vi "AAroute.vi"() -> ()   [LabVIEW 2014]
uses:
  <vilib>/Utility/sysdir.llb/System Directory Type.ctl
  <vilib>/httpClient/LabVIEWHTTPClient.lvlib
panel:
  out "time":string
  in  "저장 경로":path
  out "Distance":string="0"
  in  "?":bool
  in  "정규식 5":string
  in  "정규식 4":string
  in  "정규식 3":string
  in  "?":bool
  in  "?":bool
  out "x fmc 플랜":string
  out "FMS 플랜":string
  in  "Destination":string
  in  "departure":string
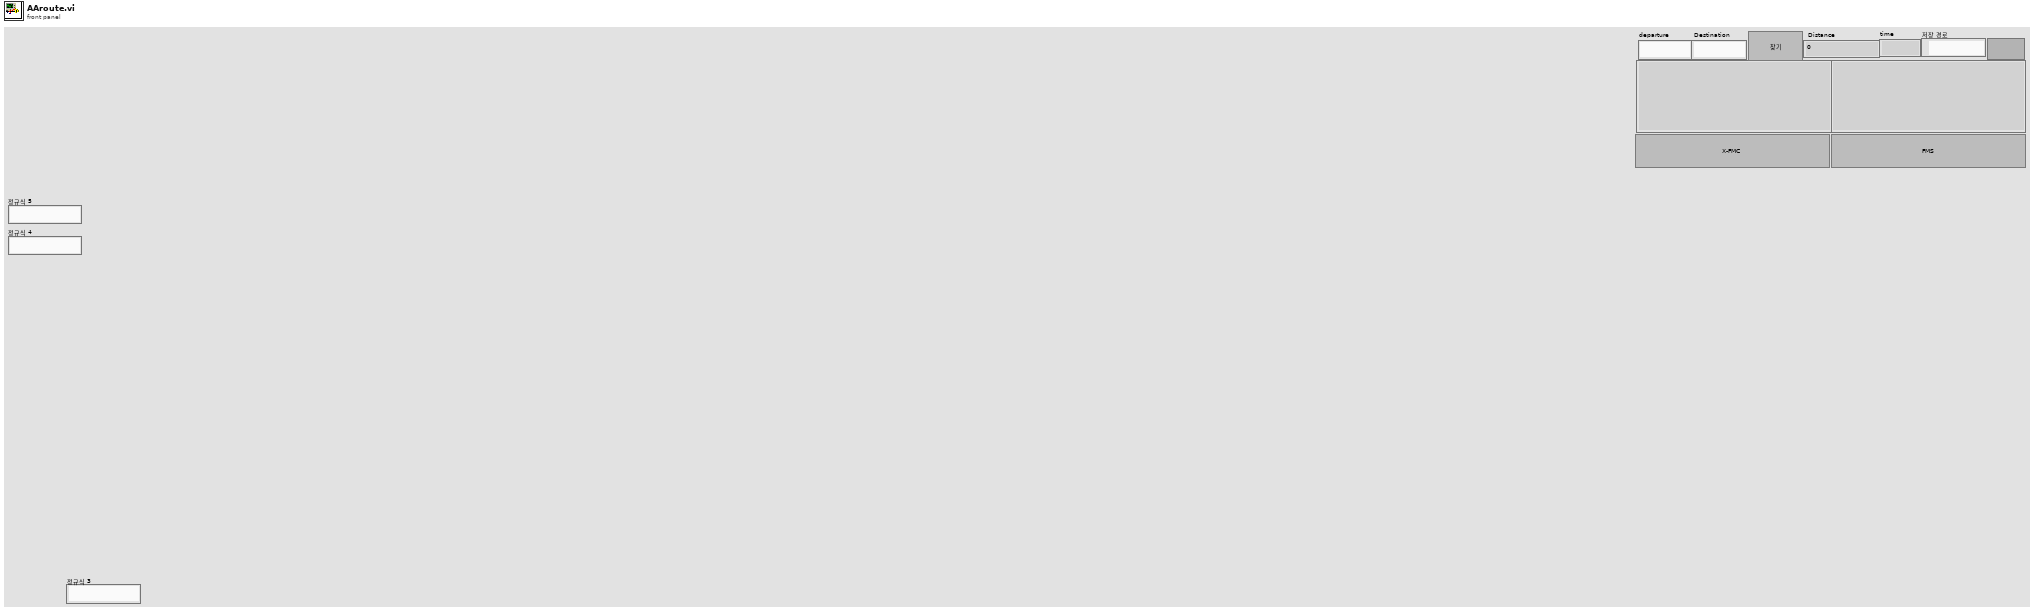
[diagram p1: front panel]
types:
  T1 = enum16{"open", "replace", "create", "open or create", "replace or create", "replace or create with confirmation"}
  T2 = typedef "System Directory Type.ctl" = i32
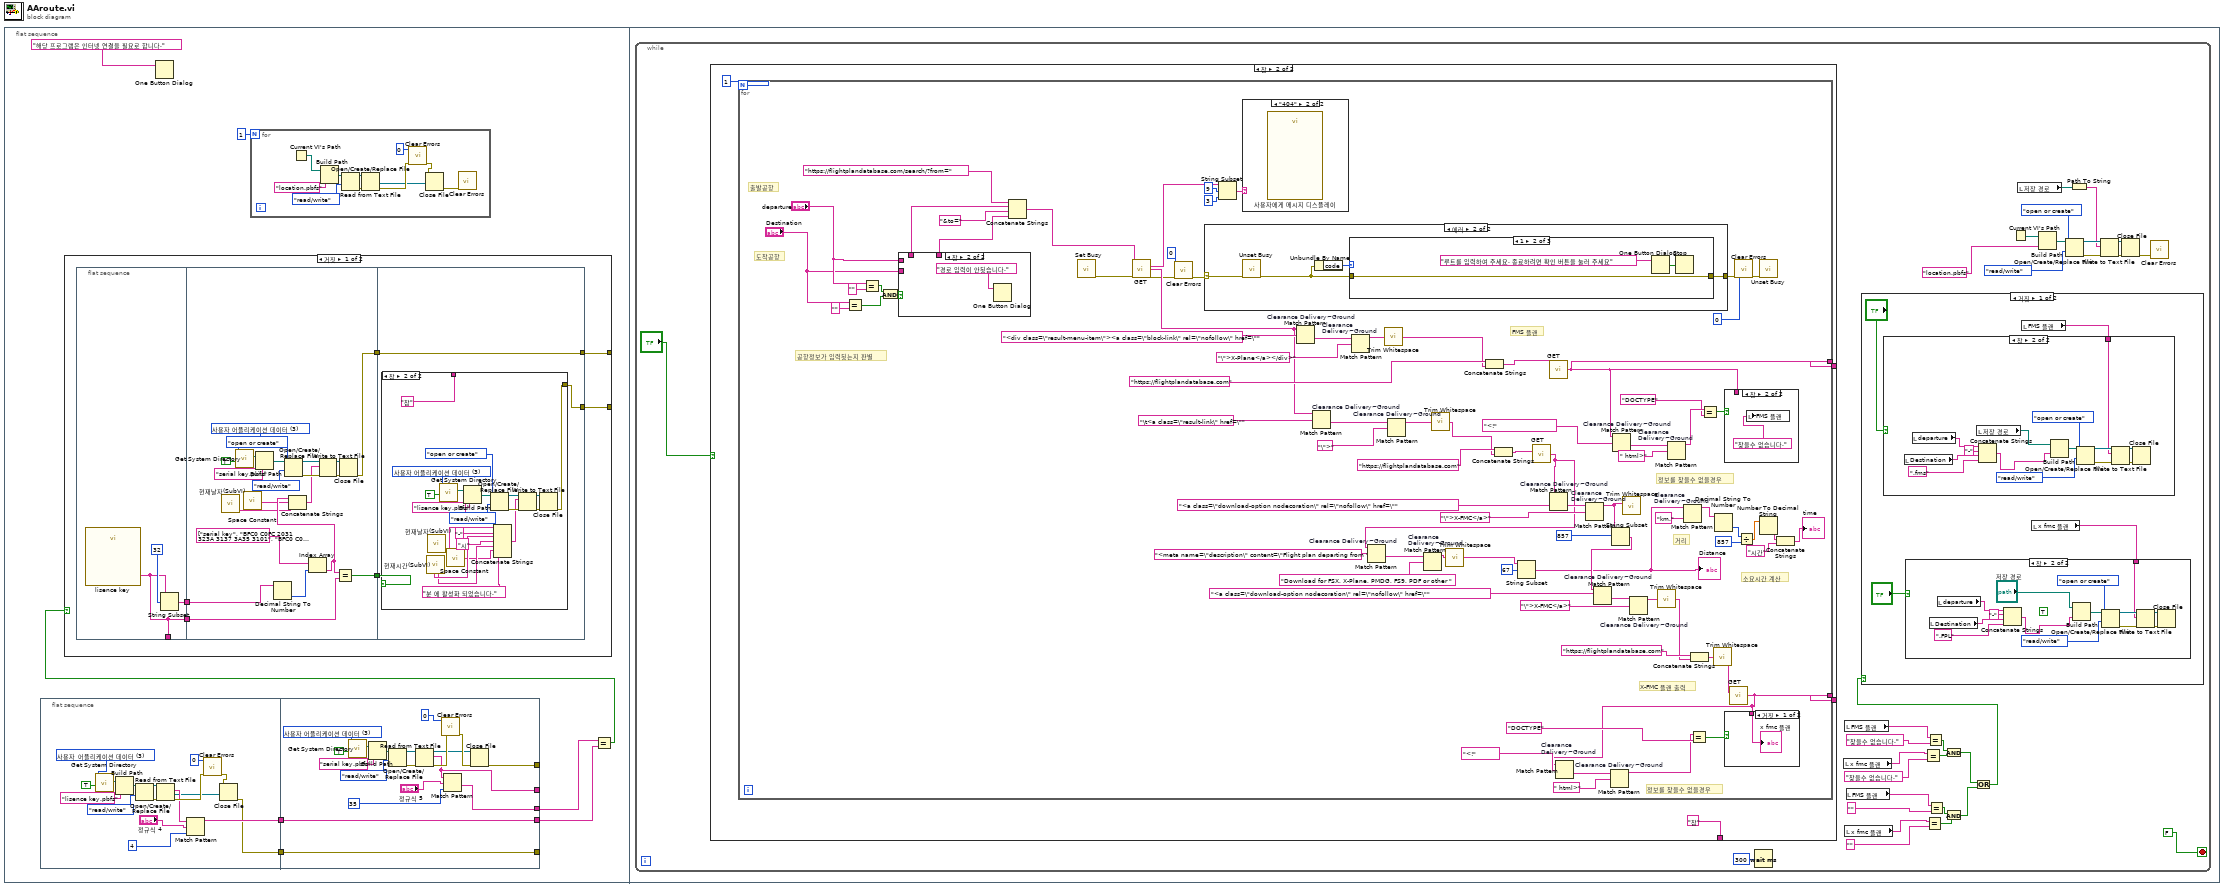
[diagram p0: block diagram]
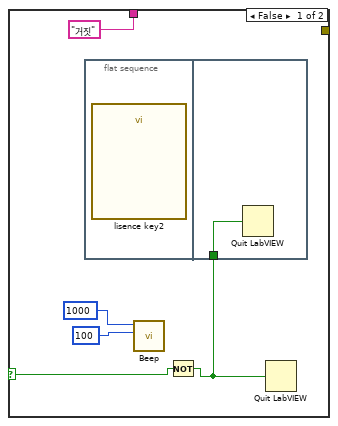
[diagram p2: hidden frame]
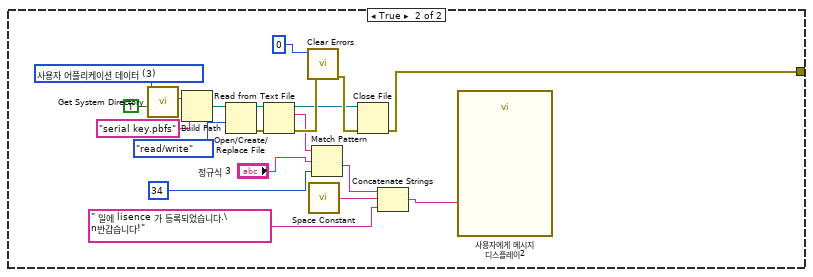
[diagram p3: hidden frame]
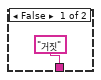
[diagram p7: hidden frame]
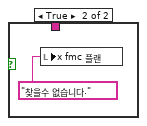
[diagram p9: hidden frame]
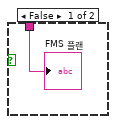
[diagram p10: hidden frame]
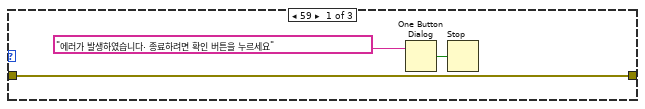
[diagram p13: hidden frame]
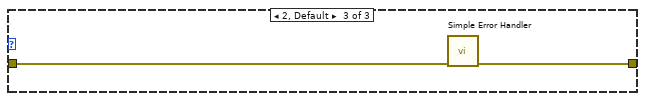
[diagram p14: hidden frame]
diagram:
  n1 = flat-sequence {
    frame #0 {
      n2 = flat-sequence {
        tunnel: [w20] -> w7
        tunnel: [w19] -> w6
        tunnel: [w42] -> w4
        tunnel: w7 -> [w42]
        tunnel: [w40] -> w5
        tunnel: [w36] -> _
        tunnel: [w38] -> _
        tunnel: w6 -> [w38]
        tunnel: [w37] -> _
        frame #0 {
          w25 = T2 3 items=["사용자 홈"=0, "사용자 데스크탑"=1, "사용자 문서"=2, "사용자 어플리케이션 데이터"=3, "사용자 환경"=4, "사용자 임시"=5, "퍼블릭 문서"=6, "퍼블릭 어플리케이션 데이터"=7, "퍼블릭 환경"=8, "퍼블릭 캐시"=13, "시스템 코어 라이브러리"=9, "시스템 설치된 라이브러리"=10, "어플리케이션 파일"=11, "부팅 볼륨 루트"=12] ("system directory type")
          n3 = call <vilib>:"Get System Directory.vi"("create directory if not found? (F)"=TRUE, "system directory type"=w25) -> ("system directory"=w24:path)  [unwired: 9 in]
          n4 = Build Path(base path=w24, name or relative path="lisence key.pbfs" ("이름 또는 상대 경로")) -> (appended path=w23:path)
          n5 = Open/Create/Replace File(file path (use dialog)=w23, access (0:read/write)=enum16{"read/write", "read-only", "write-only"}."read/write" ("접근(0:읽기/쓰기)")) -> (refnum out=w29:refnum<file>, error out=w28:errorcluster)  [unwired: 4 in, 1 out]
          n6 = Read from Text File(file (use dialog)=w29, error in=w28) -> (refnum out=w30:refnum<file>, text=w31:string, error out=w33:errorcluster)  [unwired: 2 in, 1 out]
          n7 = Match Pattern(string=w31, regular expression="정규식 4", offset (0)=4 ("오프셋(0) 2")) -> (before substring=w20:string)  [unwired: 3 out]
          n8 = call <vilib>:"Clear Errors.vi"("error in (no error)"=w33, "specific error code to clear (0: all)"=0) -> ("error out"=w34:errorcluster)  [unwired: 4 in, 1 out]
          n9 = Close File(refnum=w30, error in=w34) -> (error out=w19:errorcluster)  [unwired: 1 out]
        }
        frame #1 {
          w48 = T2 3 items=["사용자 홈"=0, "사용자 데스크탑"=1, "사용자 문서"=2, "사용자 어플리케이션 데이터"=3, "사용자 환경"=4, "사용자 임시"=5, "퍼블릭 문서"=6, "퍼블릭 어플리케이션 데이터"=7, "퍼블릭 환경"=8, "퍼블릭 캐시"=13, "시스템 코어 라이브러리"=9, "시스템 설치된 라이브러리"=10, "어플리케이션 파일"=11, "부팅 볼륨 루트"=12] ("system directory type")
          n10 = call <vilib>:"Get System Directory.vi"("create directory if not found? (F)"=TRUE, "system directory type"=w48) -> ("system directory"=w49:path)  [unwired: 9 in]
          n11 = Build Path(base path=w49, name or relative path="serial key.pbfs" ("이름 또는 상대 경로")) -> (appended path=w50:path)
          n12 = Open/Create/Replace File(file path (use dialog)=w50, access (0:read/write)=enum16{"read/write", "read-only", "write-only"}."read/write" ("접근(0:읽기/쓰기)")) -> (refnum out=w44:refnum<file>, error out=w45:errorcluster)  [unwired: 4 in, 1 out]
          n13 = Read from Text File(file (use dialog)=w44, error in=w45) -> (refnum out=w43:refnum<file>, text=w36:string, error out=w52:errorcluster)  [unwired: 2 in, 1 out]
          n14 = call <vilib>:"Clear Errors.vi"("error in (no error)"=w52, "specific error code to clear (0: all)"=0) -> ("error out"=w53:errorcluster)  [unwired: 4 in, 1 out]
          n15 = Match Pattern(string=w36, regular expression="정규식 5", offset (0)=35 ("오프셋(0)")) -> (after substring=w40:string)  [unwired: 3 out]
          n16 = Close File(refnum=w43, error in=w53) -> (error out=w37:errorcluster)  [unwired: 1 out]
        }
      }
      n17 = One Button Dialog(message="해당 프로그램은 인터넷 연결을 필요로 합니다." ("메시지")) -> ()  [unwired: 1 in, 1 out]
      n18 = for {
        N: 1 -> [_]
        n19 = Current VI's Path() -> (path=w9:path)
        n20 = Build Path(base path=w9, name or relative path="location.pbfs" ("이름 또는 상대 경로")) -> (appended path=w10:path)
        n21 = Open/Create/Replace File(file path (use dialog)=w10, access (0:read/write)=enum16{"read/write", "read-only", "write-only"}."read/write" ("접근(0:읽기/쓰기)")) -> (refnum out=w14:refnum<file>, error out=w13:errorcluster)  [unwired: 4 in, 1 out]
        n22 = Read from Text File(file (use dialog)=w14, error in=w13) -> (refnum out=w15:refnum<file>, error out=w16:errorcluster)  [unwired: 2 in, 2 out]
        n23 = call <vilib>:"Clear Errors.vi"("error in (no error)"=w16, "specific error code to clear (0: all)"=0) -> ("error out"=w17:errorcluster)  [unwired: 4 in, 1 out]
        n24 = Close File(refnum=w15, error in=w17) -> (error out=w8:errorcluster)  [unwired: 1 out]
        n25 = call <vilib>:"Clear Errors.vi"("error in (no error)"=w8) -> ()  [unwired: 5 in, 2 out]
      }
      n26 = Equal?(x=w5, y=w4) -> (x = y?=w3:bool)
      n27 = case shown="거짓" w3 {
        tunnel: [w56 w115] -> _
        tunnel: [w55 _] -> _
        frame False {
          n28 = flat-sequence {
            tunnel: [w62] -> w60
            tunnel: [w61] -> w59
            tunnel: [w61] -> _
            tunnel: w60 -> [w84]
            tunnel: [w81] -> w58
            tunnel: w59 -> [w82]
            tunnel: [w65] -> w57
            tunnel: w58 -> [w87]
            tunnel: [w86] -> w56
            tunnel: w57 -> [w85]
            tunnel: [w85] -> w55
            frame #0 {
              n29 = call "lisence key"() -> ("lisence key"=w61:string)  [unwired: 17 in, 2 out]
              n30 = String Subset(string=w61, offset (0)=32 ("오프셋(0)")) -> (substring=w62:string)  [unwired: 1 in]
            }
            frame #1 {
              w74 = T2 3 items=["사용자 홈"=0, "사용자 데스크탑"=1, "사용자 문서"=2, "사용자 어플리케이션 데이터"=3, "사용자 환경"=4, "사용자 임시"=5, "퍼블릭 문서"=6, "퍼블릭 어플리케이션 데이터"=7, "퍼블릭 환경"=8, "퍼블릭 캐시"=13, "시스템 코어 라이브러리"=9, "시스템 설치된 라이브러리"=10, "어플리케이션 파일"=11, "부팅 볼륨 루트"=12] ("system directory type")
              n31 = call "현재날자(SubVI).vi"() -> ("월,일 을 문자열로"=w69:string)  [unwired: 5 in, 6 out]
              n32 = call <vilib>:"Get System Directory.vi"("create directory if not found? (F)"=TRUE, "system directory type"=w74) -> ("system directory"=w73:path)  [unwired: 9 in]
              n33 = call <vilib>:"Space Constant.vi"() -> ("String"=w68:string)
              n34 = Build Path(base path=w73, name or relative path="serial key.pbfs" ("이름 또는 상대 경로")) -> (appended path=w72:path)
              n35 = Decimal String To Number(string=w84) -> (number=w83:i32)  [unwired: 2 in, 1 out]
              n36 = Open/Create/Replace File(file path (use dialog)=w72, operation (0:open)=T1."open or create" ("동작(0:open)"), access (0:read/write)=enum16{"read/write", "read-only", "write-only"}."read/write" ("접근(0:읽기/쓰기)")) -> (refnum out=w80:refnum<file>, error out=w79:errorcluster)  [unwired: 3 in, 1 out]
              n37 = Index Array(array=string[] ["serial key", "BFC0 C0FC 2031 323A 3137 3A35 3101", "BFC0 C0FC 2031 323A 3138 3A30 3902", "BFC0 C0FC 2031 323A 3139 3A30 3903", "BFC0 C0FC 2031 323A 3230 3A30 3904", "BFC0 C0FC 2031 323A 3231 3A30 3905", "BFC0 C0FC 2031 323A 3232 3A30 3906", "BFC0 C0FC 2031 323A 3233 3A30 3907", "BFC0 C0FC 2031 323A 3234 3A30 3908", "BFC0 C0FC 2031 323A 3235 3A30 3909", "BFC0 C0FC 2031 323A 3236 3A30 3910", "BFC0 C0FC 2031 323A 3237 3A30 3911", "BFC0 C0FC 2031 323A 3238 3A30 3912", "BFC0 C0FC 2031 323A 3239 3A30 3913", "BFC0 C0FC 2031 323A 3036 3A33 3214", "BFC0 C0FC 2031 323A 3037 3A33 3215", "BFC0 C0FC 2031 323A 3038 3A33 3216", "BFC0 C0FC 2031 323A 3038 3A33 3217", "BFC0 C0FC 2031 323A 3039 3A33 3218", "BFC0 C0FC 2031 323A 3039 3A35 3019", "BFC0 C0FC 2031 323A 3130 3A35 3020", "BFC0 C0FC 2031 323A 3131 3A35 3121", "BFC0 C8C4 2031 313A 3536 3A33 3222", "BFC0 C8C4 2031 313A 3537 3A33 3223", "BFC0 C8C4 2031 313A 3538 3A33 3224", "BFC0 C8C4 2031 313A 3539 3A33 3225", "BFC0 C0FC 2031 323A 3030 3A33 3226", "BFC0 C0FC 2031 323A 3031 3A33 3227", "BFC0 C0FC 2031 323A 3032 3A33 3228", "BFC0 C0FC 2031 323A 3033 3A33 3229", "BFC0 C0FC 2031 323A 3034 3A33 3230", "BFC0 C0FC 2031 323A 3035 3A33 3231", "BFC0 C0FC 2031 323A 3036 3A33 3232", "BFC0 C0FC 2031 323A 3037 3A33 3233", "BFC0 C0FC 2031 323A 3038 3A33 3234", "BFC0 C0FC 2033 3A34 373A 3031 0035 ", "BFC0 C0FC 2033 3A34 383A 3234 0036", "BFC0 C0FC 2033 3A34 393A 3132 0037", "BFC0 C0FC 2033 3A35 303A 3534 0038", "BFC0 C0FC 2033 3A35 313A 3231 0039 ", "BFC0 C0FC 2033 3A35 323A 3333 0040 ", "BFC0 C0FC 2033 3A35 333A 3030 0041", "BFC0 C0FC 2033 3A35 343A 3432 0042", "BFC0 C0FC 2033 3A35 353A 3431 0043", "BFC0 C0FC 2033 3A35 363A 3131 0044", "BFC0 C0FC 2033 3A35 373A 3239 0045", "BFC0 C0FC 2033 3A35 383A 3539 0046", "BFC0 C0FC 2033 3A35 393A 3533 0047", "BFC0 C0FC 2034 3A30 303A 3430 0048 "] ("출력 배열"), index=w83) -> (element=w70:string)
              n38 = Concatenate Strings(w70, w68, w69) -> (w71:string)
              n39 = Write to Text File(file (use dialog)=w80, text=w71, error in=w79) -> (refnum out=w77:refnum<file>, error out=w78:errorcluster)  [unwired: 1 in, 1 out]
              n40 = Equal?(x=w70, y=w82) -> (x = y?=w81:bool)
              n41 = Close File(refnum=w77, error in=w78) -> (error out=w65:errorcluster)  [unwired: 1 out]
            }
            frame #2 {
              n42 = case shown="참" w87 {
                selector: w87 -> [w90 _]
                tunnel: ["거짓" "참"] -> _
                tunnel: [_ w94] -> w86
                frame False {
                  n43 = flat-sequence {
                    tunnel: w91 -> [w93]
                    frame #0 {
                      n44 = call "lisence key2"() -> ()  [unwired: 10 in, 2 out]
                    }
                    frame #1 {
                      n45 = Quit LabVIEW(quit? (T)=w93) -> ()
                    }
                  }
                  n46 = call <vilib>:"Beep.vi"("duration (msec)"=u32 100, "frequency (Hz)"=u32 1000) -> ()  [unwired: 10 in]
                  n47 = Not(x=w90) -> (.not. x?=w91:bool)
                  n48 = Quit LabVIEW(quit? (T)=w91) -> ()
                }
                frame True {
                  w110 = T2 3 items=["사용자 홈"=0, "사용자 데스크탑"=1, "사용자 문서"=2, "사용자 어플리케이션 데이터"=3, "사용자 환경"=4, "사용자 임시"=5, "퍼블릭 문서"=6, "퍼블릭 어플리케이션 데이터"=7, "퍼블릭 환경"=8, "퍼블릭 캐시"=13, "시스템 코어 라이브러리"=9, "시스템 설치된 라이브러리"=10, "어플리케이션 파일"=11, "부팅 볼륨 루트"=12] ("system directory type")
                  n49 = call "현재시간(SubVI).vi"() -> ("분 문자열"=w99:string, "시 문자열"=w101:string)  [unwired: 3 in, 7 out]
                  n50 = call "현재날자(SubVI).vi"() -> ("월,일 을 문자열로"=w103:string)  [unwired: 5 in, 6 out]
                  n51 = call <vilib>:"Get System Directory.vi"("create directory if not found? (F)"=TRUE, "system directory type"=w110) -> ("system directory"=w111:path)  [unwired: 9 in]
                  n52 = call <vilib>:"Space Constant.vi"() -> ("String"=w98:string)
                  n53 = Build Path(base path=w111, name or relative path="lisence key.pbfs" ("이름 또는 상대 경로")) -> (appended path=w112:path)
                  n54 = Open/Create/Replace File(file path (use dialog)=w112, operation (0:open)=T1."open or create" ("동작(0:open)"), access (0:read/write)=enum16{"read/write", "read-only", "write-only"}."read/write" ("접근(0:읽기/쓰기)")) -> (refnum out=w108:refnum<file>, error out=w106:errorcluster)  [unwired: 3 in, 1 out]
                  n55 = Concatenate Strings(w103, "-", w101, "시", w99, w98, "분 에 활성화 되었습니다.") -> (w104:string)
                  n56 = Write to Text File(file (use dialog)=w108, text=w104, error in=w106) -> (refnum out=w109:refnum<file>, error out=w105:errorcluster)  [unwired: 1 in, 1 out]
                  n57 = Close File(refnum=w109, error in=w105) -> (error out=w94:errorcluster)  [unwired: 1 out]
                }
              }
            }
          }
        }
        frame True {
          w128 = T2 3 items=["사용자 홈"=0, "사용자 데스크탑"=1, "사용자 문서"=2, "사용자 어플리케이션 데이터"=3, "사용자 환경"=4, "사용자 임시"=5, "퍼블릭 문서"=6, "퍼블릭 어플리케이션 데이터"=7, "퍼블릭 환경"=8, "퍼블릭 캐시"=13, "시스템 코어 라이브러리"=9, "시스템 설치된 라이브러리"=10, "어플리케이션 파일"=11, "부팅 볼륨 루트"=12] ("system directory type")
          n58 = call <vilib>:"Get System Directory.vi"("create directory if not found? (F)"=TRUE, "system directory type"=w128) -> ("system directory"=w129:path)  [unwired: 9 in]
          n59 = Build Path(base path=w129, name or relative path="serial key.pbfs" ("이름 또는 상대 경로")) -> (appended path=w130:path)
          n60 = Open/Create/Replace File(file path (use dialog)=w130, access (0:read/write)=enum16{"read/write", "read-only", "write-only"}."read/write" ("접근(0:읽기/쓰기)")) -> (refnum out=w124:refnum<file>, error out=w125:errorcluster)  [unwired: 4 in, 1 out]
          n61 = Read from Text File(file (use dialog)=w124, error in=w125) -> (refnum out=w123:refnum<file>, text=w131:string, error out=w133:errorcluster)  [unwired: 2 in, 1 out]
          n62 = call <vilib>:"Clear Errors.vi"("error in (no error)"=w133, "specific error code to clear (0: all)"=0) -> ("error out"=w134:errorcluster)  [unwired: 4 in, 1 out]
          n63 = call <vilib>:"Space Constant.vi"() -> ("String"=w117:string)
          n64 = Match Pattern(string=w131, regular expression="정규식 3", offset (0)=34 ("오프셋(0)")) -> (after substring=w120:string)  [unwired: 3 out]
          n65 = Close File(refnum=w123, error in=w134) -> (error out=w115:errorcluster)  [unwired: 1 out]
          n66 = Concatenate Strings(w120, w117, " 일에 lisence 가 등록되었습니다.\n반갑습니다!" ("Message")) -> (w119:string)
          n67 = call "사용자에게 메시지 디스플레이2"("Message"=w119) -> ()  [unwired: 9 in, 2 out]
        }
      }
    }
    frame #1 {
      n68 = while {
        stop <- FALSE stop-if-true
        n69 = case shown="참" "?" {
          tunnel: [_ w201] -> _
          tunnel: [_ w200] -> _
          tunnel: ["거짓" "참"] -> _
          frame False {
          }
          frame True {
            n70 = for {
              N: 1 -> [_]
              tunnel: [w224] -> w201
              tunnel: [w223] -> w200
              # "FMS 플랜"
              # "거리"
              # "소요시간 계산"
              # "X-FMC 플랜 출력"
              # "정보를 찾을수 없을경우"
              # "정보를 찾을수 없을경우"
              # "공항정보가 입력됫는지 판별"
              # "도착공항"
              # "출발공항"
              n71 = Equal?(x="Destination", y="") -> (x = y?=w211:bool)
              n72 = Equal?(x="departure", y="") -> (x = y?=w213:bool)
              n73 = And(x=w213, y=w211) -> (x .and. y?=w214:bool)
              n74 = case shown="참" w214 {
                tunnel: "departure" -> [w285 _]
                tunnel: "Destination" -> [w284 _]
                tunnel: [w285 _] -> w207
                tunnel: [w284 _] -> w206
                frame False {
                }
                frame True {
                  n75 = One Button Dialog(message="경로 입력이 안됫습니다." ("메시지")) -> ()  [unwired: 1 in, 1 out]
                }
              }
              n76 = Concatenate Strings("https://flightplandatabase.com/search/?from=" ("문자열"), w207, "&to=" ("문자열"), w206) -> (w274:string)
              n77 = call <vilib>:"Set Busy.vi"() -> ("error out"=w279:errorcluster)  [unwired: 10 in, 1 out]
              n78 = call <vilib>:"GET.vi"("url"=w274, "error in (no error)"=w279) -> ("headers"=w283:string, "body"=w243:string, "error out"=w219:errorcluster)  [unwired: 10 in, 1 out]
              n79 = call <vilib>:"Clear Errors.vi"("error in (no error)"=w219, "specific error code to clear (0: all)"=0) -> ("error out"=w220:errorcluster)  [unwired: 4 in, 1 out]
              n80 = case shown="에러" w220 {
                selector: w220 -> [w291 w294]
                tunnel: [w291 w292] -> w216
                frame No Error {
                }
                frame Error {
                  n81 = call <vilib>:"Unset Busy.vi"("error in (no error)"=w294) -> ("error out"=w293:errorcluster)  [unwired: 10 in]
                  n82 = Unbundle By Name(w293) -> ("code"=w295:i32)
                  n83 = case shown="1" w295 {
                    tunnel: w293 -> [w296 w301 w303]
                    tunnel: [w296 w301 w302] -> w292
                    frame 59 {
                      n84 = One Button Dialog(message="에러가 발생하였습니다. 종료하려면 확인 버튼을 누르세요" ("메시지")) -> (true=w297:bool)  [unwired: 1 in]
                      n85 = Stop(stop? (T)=w297) -> ()
                    }
                    frame 1 {
                      n86 = One Button Dialog(message="루트를 입력하여 주세요. 종료하려면 확인 버튼을 눌러 주세요" ("메시지")) -> (true=w299:bool)  [unwired: 1 in]
                      n87 = Stop(stop? (T)=w299) -> ()
                    }
                    frame 2, Default {
                      n88 = call <vilib>:"Simple Error Handler.vi"("error in (no error)"=w303) -> ("error out"=w302:errorcluster)  [unwired: 4 in, 4 out]
                    }
                  }
                }
              }
              n89 = String Subset(string=w283, offset (0)=9 ("오프셋(0)"), length (rest)=3 ("길이(나머지)")) -> (substring=w280:string)
              n90 = case shown="\"404\"" w280 {
                frame "거짓", Default {
                }
                frame "404" {
                  n91 = call "사용자에게 메시지 디스플레이"() -> ()  [unwired: 10 in, 2 out]
                }
              }
              n92 = Match Pattern "Clearance Delivery~Ground"(string=w243, regular expression="<div class=\"result-menu-item\"><a class=\"block-link\" rel=\"nofollow\" href=\"" ("정규식")) -> (after substring=w277:string)  [unwired: 1 in, 3 out]
              n93 = Match Pattern "Clearance Delivery~Ground"(string=w243, regular expression="\t<a class=\"result-link\" href=\"" ("정규식")) -> (after substring=w268:string)  [unwired: 1 in, 3 out]
              n94 = Match Pattern "Clearance Delivery~Ground"(string=w277, regular expression="\">X-Plane</a></div>" ("정규식")) -> (before substring=w275:string)  [unwired: 1 in, 3 out]
              n95 = call <vilib>:"Trim Whitespace.vi"("string"=w275) -> ("trimmed string"=w269:string)  [unwired: 1 in]
              n96 = Match Pattern "Clearance Delivery~Ground"(string=w268, regular expression="\">" ("정규식")) -> (before substring=w265:string)  [unwired: 1 in, 3 out]
              n97 = call <vilib>:"Trim Whitespace.vi"("string"=w265) -> ("trimmed string"=w263:string)  [unwired: 1 in]
              n98 = Concatenate Strings("https://flightplandatabase.com" ("url"), w269) -> (w270:string)
              n99 = Concatenate Strings("https://flightplandatabase.com" ("url"), w263) -> (w260:string)
              n100 = call <vilib>:"GET.vi"("url"=w260) -> ("body"=w241:string)  [unwired: 11 in, 3 out]
              n101 = Match Pattern "Clearance Delivery~Ground"(string=w241, regular expression="<meta name=\"description\" content=\"Flight plan departing from " ("정규식")) -> (after substring=w244:string)  [unwired: 1 in, 3 out]
              n102 = Match Pattern "Clearance Delivery~Ground"(string=w244, regular expression="Download for FSX, X-Plane, PMDG, FS9, PDF or other " ("정규식")) -> (before substring=w246:string)  [unwired: 1 in, 3 out]
              n103 = call <vilib>:"Trim Whitespace.vi"("string"=w246) -> ("trimmed string"=w240:string)  [unwired: 1 in]
              n104 = String Subset(string=w240, offset (0)=67 ("오프셋(0)")) -> (substring=w227:string)  [unwired: 1 in]
              "Distance" <- w227
              n105 = call <vilib>:"GET.vi"("url"=w270) -> ("body"=w223:string)  [unwired: 11 in, 3 out]
              n106 = Match Pattern "Clearance Delivery~Ground"(string=w241, regular expression="<a class=\"download-option nodecoration\" rel=\"nofollow\" href=\"" ("정규식")) -> (after substring=w259:string)  [unwired: 1 in, 3 out]
              n107 = Match Pattern "Clearance Delivery~Ground"(string=w259, regular expression="\">X-FMC</a>" ("정규식")) -> (before substring=w258:string)  [unwired: 1 in, 3 out]
              n108 = String Subset(string=w258, offset (0)=857 ("길이(나머지)")) -> (substring=w252:string)  [unwired: 1 in]
              n109 = Match Pattern "Clearance Delivery~Ground"(string=w252, regular expression="<a class=\"download-option nodecoration\" rel=\"nofollow\" href=\"" ("정규식")) -> (after substring=w254:string)  [unwired: 1 in, 3 out]
              n110 = Match Pattern "Clearance Delivery~Ground"(string=w223, regular expression="<!" ("문자열")) -> (after substring=w237:string)  [unwired: 1 in, 3 out]
              n111 = call <vilib>:"Trim Whitespace.vi"("string"=w258) -> ()  [unwired: 1 in, 1 out]
              n112 = Match Pattern "Clearance Delivery~Ground"(string=w254, regular expression="\">X-FMC</a>" ("정규식")) -> (before substring=w253:string)  [unwired: 1 in, 3 out]
              n113 = call <vilib>:"Trim Whitespace.vi"("string"=w253) -> ("trimmed string"=w250:string)  [unwired: 1 in]
              n114 = Match Pattern "Clearance Delivery~Ground"(string=w237, regular expression=" html>" ("정규식")) -> (before substring=w236:string)  [unwired: 1 in, 3 out]
              n115 = Match Pattern "Clearance Delivery~Ground"(string=w227, regular expression="km." ("정규식")) -> (before substring=w225:string)  [unwired: 1 in, 3 out]
              n116 = Concatenate Strings("https://flightplandatabase.com" ("url"), w250) -> (w249:string)
              n117 = Equal?(x=w236, y="DOCTYPE") -> (x = y?=w248:bool)
              n118 = call <vilib>:"Trim Whitespace.vi"("string"=w249) -> ("trimmed string"=w229:string)  [unwired: 1 in]
              n119 = Decimal String To Number(string=w225) -> (number=w222:i32)  [unwired: 2 in, 1 out]
              n120 = case shown="참" w248 {
                tunnel: w223 -> [w289 _]
                frame False {
                  "FMS 플랜" <- w289
                }
                frame True {
                  n121 = local write "FMS 플랜"("찾을수 없습니다.") -> ()
                }
              }
              n122 = call <vilib>:"GET.vi"("url"=w229) -> ("body"=w224:string)  [unwired: 11 in, 3 out]
              n123 = Match Pattern "Clearance Delivery~Ground"(string=w224, regular expression="<!" ("문자열")) -> (after substring=w234:string)  [unwired: 1 in, 3 out]
              n124 = Match Pattern "Clearance Delivery~Ground"(string=w234, regular expression=" html>" ("정규식")) -> (before substring=w231:string)  [unwired: 1 in, 3 out]
              n125 = Equal?(x=w231, y="DOCTYPE") -> (x = y?=w247:bool)
              n126 = case shown="거짓" w247 {
                tunnel: w224 -> [w287 _]
                frame False {
                  "x fmc 플랜" <- w287
                }
                frame True {
                  n127 = local write "x fmc 플랜"("찾을수 없습니다.") -> ()
                }
              }
              n128 = call <vilib>:"Clear Errors.vi"("error in (no error)"=w216, "specific error code to clear (0: all)"=0) -> ("error out"=w217:errorcluster)  [unwired: 4 in, 1 out]
              n129 = Divide(x=w222, y=857) -> (x/y=w205:dbl)
              n130 = call <vilib>:"Unset Busy.vi"("error in (no error)"=w217) -> ()  [unwired: 10 in, 1 out]
              n131 = Number To Decimal String(number=w205) -> (decimal integer string=w203:string)  [unwired: 1 in]
              n132 = Concatenate Strings(w203, "시간") -> (→"time":string)
            }
          }
        }
        n133 = Wait (ms)(milliseconds to wait=u32 300 ("대기 시간(ms)")) -> ()  [unwired: 1 out]
        n134 = local read "x fmc 플랜"() -> (w159:string)
        n135 = local read "FMS 플랜"() -> (w157:string)
        n136 = local read "x fmc 플랜"() -> (w152:string)
        n137 = local read "FMS 플랜"() -> (w154:string)
        n138 = Equal?(x=w159, y="찾을수 없습니다.") -> (x = y?=w160:bool)
        n139 = Equal?(x=w152, y="") -> (x = y?=w151:bool)
        n140 = Equal?(x=w157, y="찾을수 없습니다.") -> (x = y?=w161:bool)
        n141 = Equal?(x=w154, y="") -> (x = y?=w150:bool)
        n142 = And(x=w161, y=w160) -> (x .and. y?=w148:bool)
        n143 = And(x=w150, y=w151) -> (x .and. y?=w149:bool)
        n144 = Or(x=w148, y=w149) -> (x .or. y?=w147:bool)
        n145 = case shown="거짓" w147 {
          frame False {
            n146 = local read "FMS 플랜"() -> (w166:string)
            n147 = case shown="참" "?" {
              tunnel: w166 -> [_ w172]
              frame False {
              }
              frame True {
                n148 = local read "Destination"() -> (w175:string)
                n149 = local read "departure"() -> (w176:string)
                n150 = local read "저장 경로"() -> (w169:path)
                n151 = Concatenate Strings(w176, "-" ("문자열"), w175, ".fms" ("문자열")) -> (w170:string)
                n152 = Build Path(base path=w169, name or relative path=w170) -> (appended path=w178:path)
                n153 = Open/Create/Replace File(file path (use dialog)=w178, operation (0:open)=T1."open or create" ("동작(0:open)"), access (0:read/write)=enum16{"read/write", "read-only", "write-only"}."read/write" ("접근(0:읽기/쓰기)")) -> (refnum out=w182:refnum<file>, error out=w181:errorcluster)  [unwired: 3 in, 1 out]
                n154 = Write to Text File(file (use dialog)=w182, text=w172, error in=w181) -> (refnum out=w179:refnum<file>, error out=w180:errorcluster)  [unwired: 1 in, 1 out]
                n155 = Close File(refnum=w179, error in=w180) -> ()  [unwired: 2 out]
              }
            }
            n156 = local read "x fmc 플랜"() -> (w167:string)
            n157 = case shown="참" "?" {
              tunnel: w167 -> [_ w185]
              frame False {
              }
              frame True {
                (unwired) TRUE ("create directory if not found? (F)")
                n158 = local read "Destination"() -> (w189:string)
                n159 = local read "departure"() -> (w190:string)
                n160 = Concatenate Strings(w190, "-" ("문자열"), w189, ".FPL" ("문자열")) -> (w186:string)
                n161 = Build Path(base path="저장 경로", name or relative path=w186) -> (appended path=w192:path)
                n162 = Open/Create/Replace File(file path (use dialog)=w192, operation (0:open)=T1."open or create" ("동작(0:open)"), access (0:read/write)=enum16{"read/write", "read-only", "write-only"}."read/write" ("접근(0:읽기/쓰기)")) -> (refnum out=w196:refnum<file>, error out=w195:errorcluster)  [unwired: 3 in, 1 out]
                n163 = Write to Text File(file (use dialog)=w196, text=w185, error in=w195) -> (refnum out=w193:refnum<file>, error out=w194:errorcluster)  [unwired: 1 in, 1 out]
                n164 = Close File(refnum=w193, error in=w194) -> ()  [unwired: 2 out]
              }
            }
          }
          frame True {
          }
        }
        n165 = Current VI's Path() -> (path=w136:path)
        n166 = local read "저장 경로"() -> (w138:path)
        n167 = Build Path(base path=w136, name or relative path="location.pbfs" ("문자열")) -> (appended path=w142:path)
        n168 = Open/Create/Replace File(file path (use dialog)=w142, operation (0:open)=T1."open or create" ("동작(0:open)"), access (0:read/write)=enum16{"read/write", "read-only", "write-only"}."read/write" ("접근(0:읽기/쓰기)")) -> (refnum out=w146:refnum<file>, error out=w145:errorcluster)  [unwired: 3 in, 1 out]
        n169 = Path To String(path=w138) -> (string=w137:string)
        n170 = Write to Text File(file (use dialog)=w146, text=w137, error in=w145) -> (refnum out=w143:refnum<file>, error out=w144:errorcluster)  [unwired: 1 in, 1 out]
        n171 = Close File(refnum=w143, error in=w144) -> (error out=w135:errorcluster)  [unwired: 1 out]
        n172 = call <vilib>:"Clear Errors.vi"("error in (no error)"=w135) -> ()  [unwired: 5 in, 2 out]
      }
    }
  }
